vi "ParseIssueNumber.vi"(11 "String In":string) -> (2 "Issue":string, 3 "Series":string)   [LabVIEW 2022 SP3]
uses:
  <vilib>/Utility/error.llb/Trim Whitespace One-Sided.vi
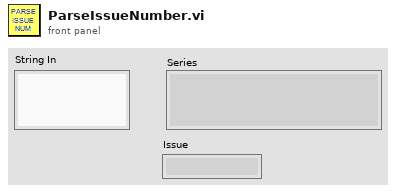
[diagram p1: front panel]
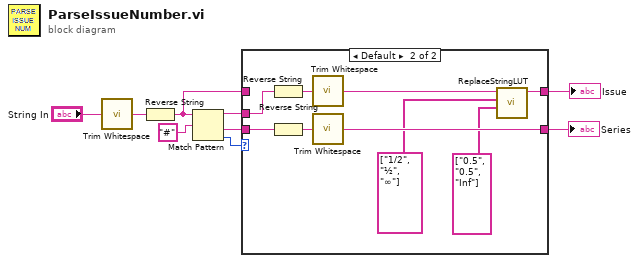
[diagram p0: block diagram]
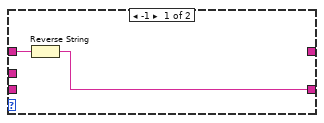
[diagram p2: hidden frame]
diagram:
  n1 = call <vilib>:"Trim Whitespace.vi"("string"="String In") -> ("trimmed string"=w1:string)  [unwired: 1 in]
  n2 = Reverse String(1:w1) -> (0:w9:string)
  n3 = Match Pattern(string=w9, regular expression="#") -> (before substring=w6:string, after substring=w7:string, offset past match=w8:i32)  [unwired: 1 in, 1 out]
  n4 = case shown="Default" w8 {
    tunnel: w6 -> [_ w20]
    tunnel: w7 -> [_ w19]
    tunnel: [_ w14] -> w5
    tunnel: [w10 w18] -> w4
    tunnel: w9 -> [w11 _]
    frame -1 {
      n5 = Reverse String(1:w11) -> (0:w10:string)
    }
    frame Default {
      n6 = Reverse String(1:w20) -> (0:w16:string)
      n7 = Reverse String(1:w19) -> (0:w17:string)
      n8 = call <vilib>:"Trim Whitespace.vi"("string"=w16) -> ("trimmed string"=w15:string)  [unwired: 1 in]
      n9 = call <vilib>:"Trim Whitespace.vi"("string"=w17) -> ("trimmed string"=w18:string)  [unwired: 1 in]
      n10 = call "ReplaceStringLUT.vi"("Replacement"=string[] ["0.5", "0.5", "Inf"], "Search List"=string[] ["1/2", "½", "∞"], "String In"=w15) -> ("String Out"=w14:string)  [unwired: 8 in]
    }
  }
  "Issue" <- w5
  "Series" <- w4
